vi "Points to ROI.vi"(8 "error in (no error)":errorcluster, 10 "Point_array":i32[](array[numeric]), 11 "Contour Type":i32=3) -> (0 "error out":errorcluster, 3 "ROI":T1)   [LabVIEW 2020]
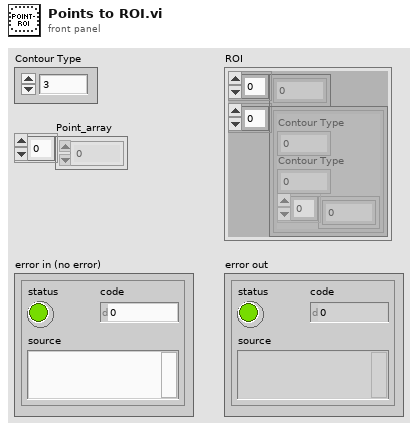
[diagram p1: front panel]
types:
  T1 = cluster{i32[], cluster{"Contour Type":u32, "Contour Type":i32, i32[]}[]}
  T2 = cluster{"Contour Type":u32, "Contour Type":i32, "Point_array":i32[]}
  T3 = cluster{"Contour Type":u32, "Contour Type":i32, "Point_array":i32[]}[]
  T4 = cluster{"Point_array":i32[], cluster{"Contour Type":u32, "Contour Type":i32, "Point_array":i32[]}[]}
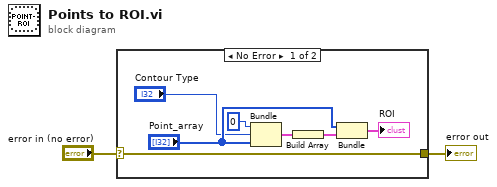
[diagram p0: block diagram]
diagram:
  n1 = case shown="No Error" "error in (no error)" {
    selector: "error in (no error)" -> [w3 w10]
    tunnel: [w3 w10] -> w2
    frame No Error {
      n2 = Bundle("Contour Type"=u32 0, "Contour Type"="Contour Type", "Point_array"="Point_array") -> (w7:T2)  [unwired: 1 in]
      n3 = Build Array(w7) -> (w8:T3)
      n4 = Bundle("Point_array"="Point_array", w8) -> (→"ROI":T4)  [unwired: 1 in]
    }
    frame Error {
    }
  }
  "error out" <- w2
